vi "Event Structure Numeric 3.vi"() -> ()   [LabVIEW 2020]
panel:
  out "NewVal":dbl
  in  "Numeric":dbl
  in  "Stop":bool
  # "Event Structure Numeric"
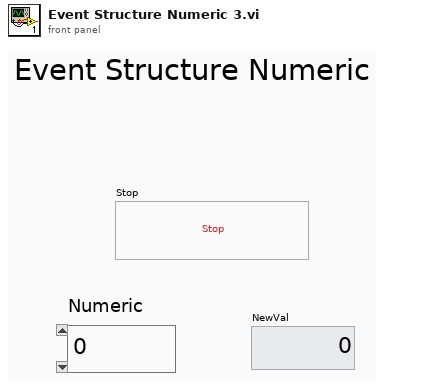
[diagram p1: front panel]
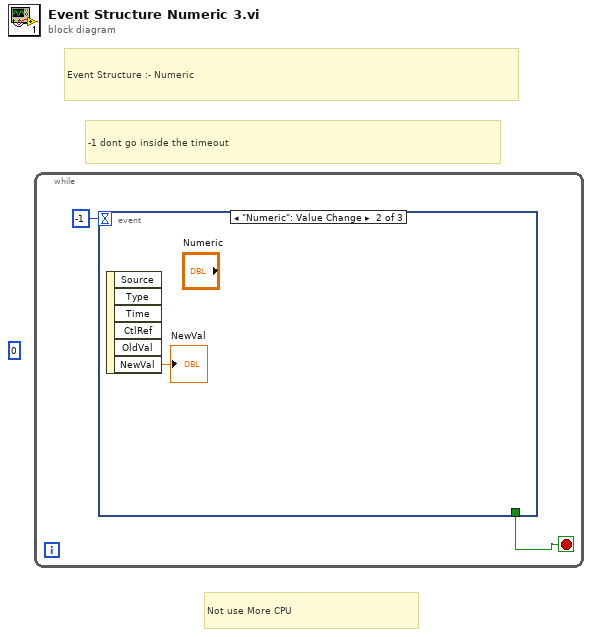
[diagram p0: block diagram]
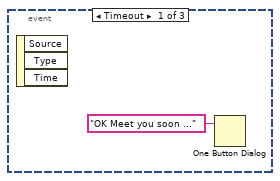
[diagram p2: hidden frame]
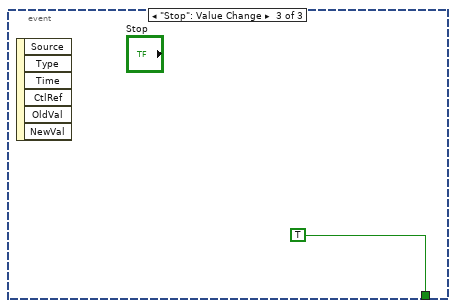
[diagram p3: hidden frame]
diagram:
  (unwired) 0
  # "Not use More CPU"
  # "-1 dont go inside the timeout"
  # "Event Structure :- Numeric"
  n1 = while {
    stop <- w1 stop-if-true
    n2 = event shown="[1] \"Numeric\": Value Change" {
      selector: _ -> [_ _ _]
      dyn-events: _ -> [_ _ _]
      timeout: -1 -> [_ _ _]
      tunnel: [_ _ TRUE] -> w1
      event Timeout {
        n3 = event-data() -> ()  [unwired: 1 in, 3 out]
        n4 = One Button Dialog(message="OK Meet you soon ...") -> ()  [unwired: 1 in, 1 out]
      }
      event "Numeric": Value Change {
        n5 = event-data() -> ("NewVal"=→"NewVal":dbl)  [unwired: 1 in, 5 out]
      }
      event "Stop": Value Change {
        n6 = event-data() -> ()  [unwired: 1 in, 6 out]
      }
    }
  }
